vi "Generador_Entorno(SubVi).vi"(9 "Objetos":path=path "C:/Users/LuisFernando/Documents/UPIITA/8vo semestre/Instrumentacion Virtual Aplicada/Solidworks/2_Ejes_Figuras/Figuras", 10 "Mundo":path=path "C:/Users/LuisFernando/Documents/UPIITA/8vo semestre/Instrumentacion Virtual Aplicada/Solidworks/2_Ejes_Figuras/Mundo.wrl", 11 "Cluster Inicial":T1={"Opción X"=0, "Opción Y"=0, "Opción Z"=0, "Posición X"=0.0, "Velocidad X"=0.0, "Posición Y"=0.0, "Velocidad Y"=0.0, "Posición Z"=0.0, "Velocidad Z"=0.0, "Escala"=[[1.0, 1.0, 1.0], [1.0, 1.0, 1.0], [1.0, 1.0, 1.0]], "Translación"=[[1.0, 1.0, 0.0], [0.0, 0.0, 0.0], [0.0, 0.0, 0.0]], "Rotación"=[[1.0, 0.0, 0.0, 0.0], [1.0, 0.0, 0.0, 0.0], [1.0, 0.0, 0.0, 0.0]], "Operacion SX"=enum."Escala", "Eje de la Figura SX"=enum."X", "Figura Geométrica SX"=enum."Cono", "Operacion SY"=enum."Escala", "Eje de la Figura SY"=enum."Y", "Figura Geométrica SY"=enum."Cono", "Operacion SZ"=enum."Escala", "Eje de la Figura SZ"=enum."Z", "Figura Geométrica SZ"=enum."Cono"}) -> (3 "3D Picture":refnum<vi>(3d-picture))   [LabVIEW 2017]
uses:
  2_Ejes_Figuras/Control_Opciones.ctl
  2_Ejes_Figuras/Control_Operacion.ctl
  2_Ejes_Figuras/Control_Eje_Figura.ctl
  2_Ejes_Figuras/Control_Figura.ctl
  <vilib>/picture/3D Picture Control/NI_3D Picture Control.lvlib
panel:
  in  "Stop Button":bool
  out "Archivos":i32
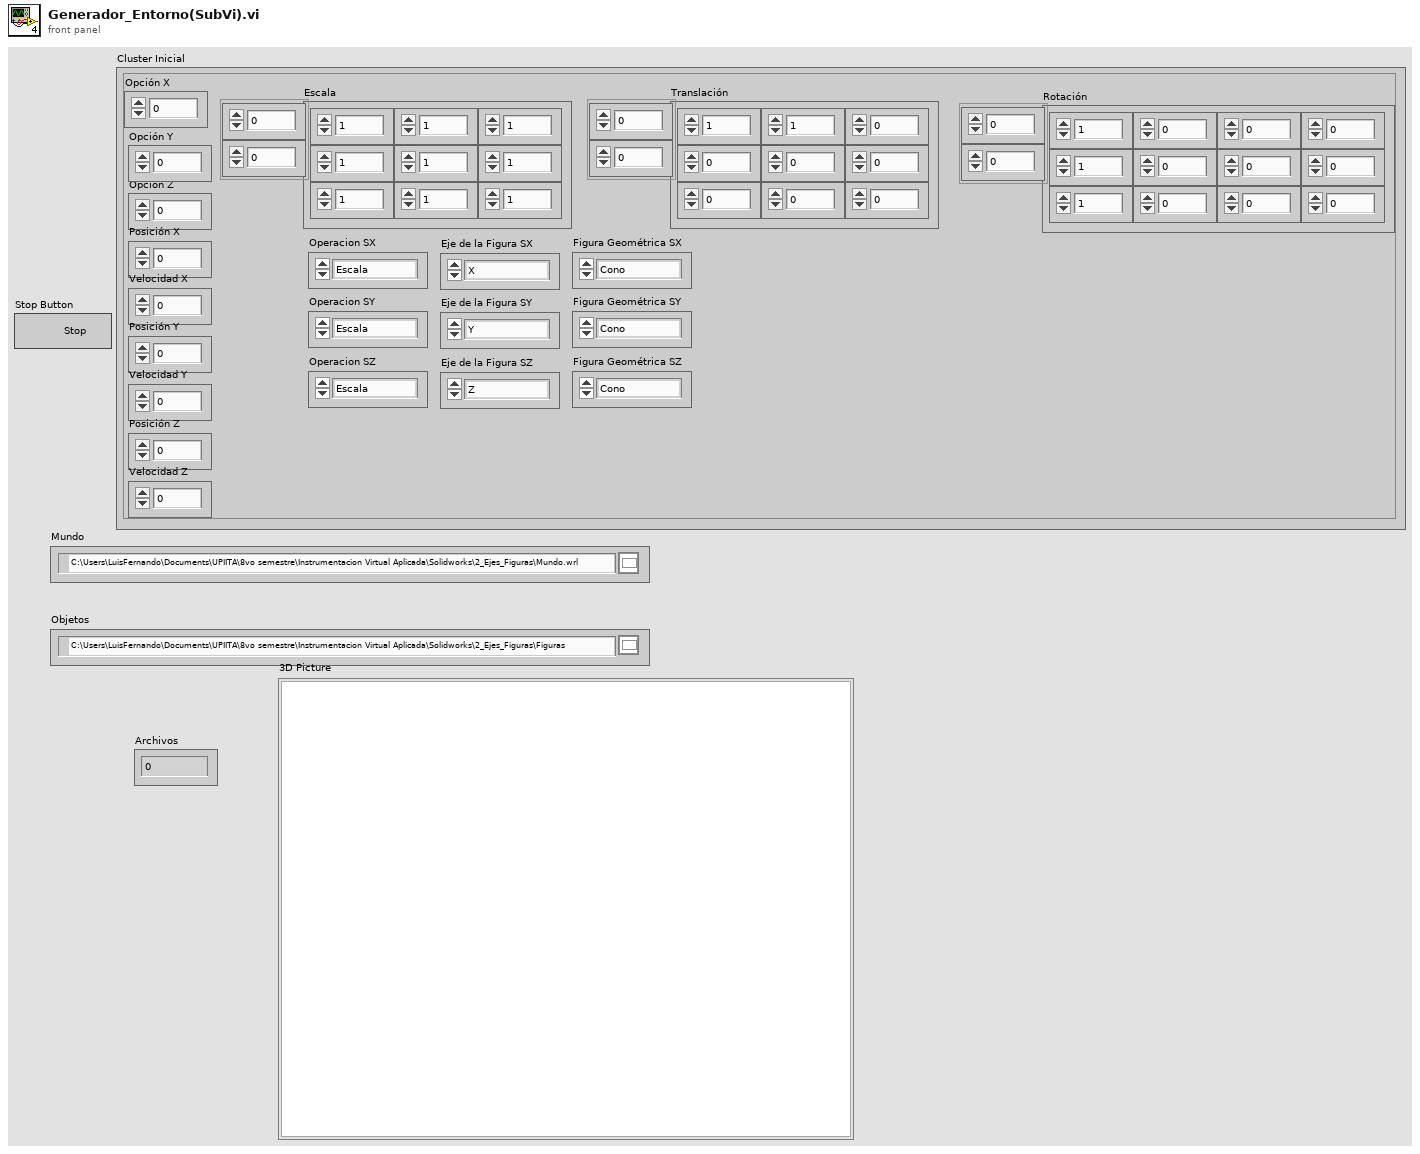
[diagram p1: front panel]
types:
  T1 = typedef "Control_Opciones.ctl" = cluster{"Opción X":i32, "Opción Y":i32, "Opción Z":i32, "Posición X":dbl, "Velocidad X":dbl, "Posición Y":dbl, "Velocidad Y":dbl, "Posición Z":dbl, "Velocidad Z":dbl, "Escala":dbl[][], "Translación":dbl[][], "Rotación":dbl[][], "Operacion SX":T2, "Eje de la Figura SX":T3, "Figura Geométrica SX":T4, "Operacion SY":T2, "Eje de la Figura SY":T3, "Figura Geométrica SY":T4, "Operacion SZ":T2, "Eje de la Figura SZ":T3, "Figura Geométrica SZ":T4}
  T2 = typedef "Control_Operacion.ctl" = enum16{"Escala", "Translación", "Rotación"}
  T3 = typedef "Control_Eje_Figura.ctl" = enum16{"X", "Y", "Z"}
  T4 = typedef "Control_Figura.ctl" = enum16{"Cono", "Esfera", "Cilindro"}
  T5 = enum16{"open", "replace", "create", "open or create", "replace or create", "replace or create with confirmation"}
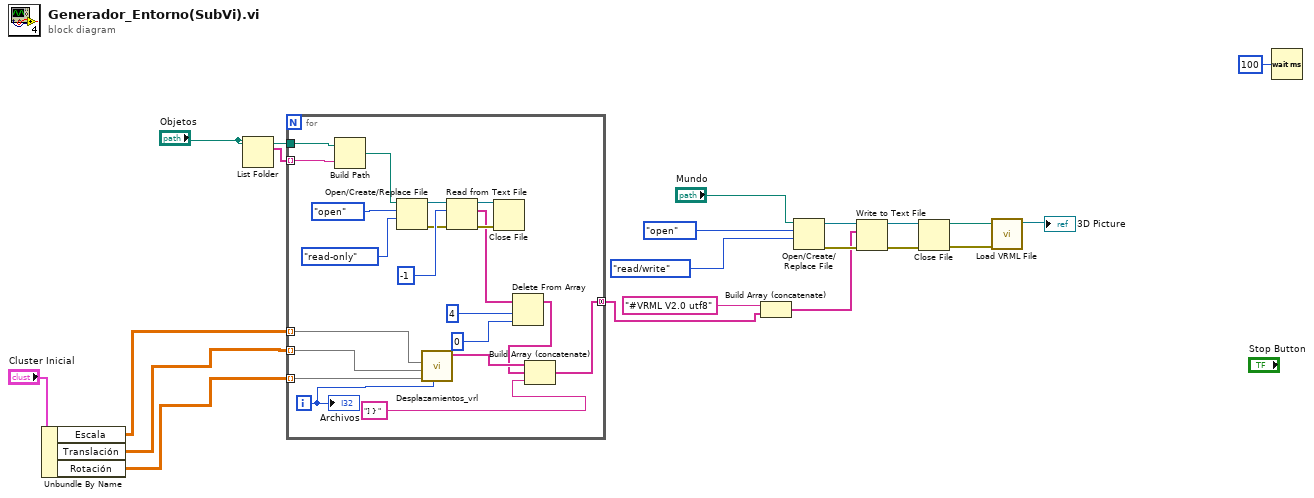
[diagram p0: block diagram]
diagram:
  n1 = Unbundle By Name("Cluster Inicial") -> ("Escala"=w3:dbl[][], "Translación"=w2:dbl[][], "Rotación"=w1:dbl[][])
  n2 = List Folder(path="Objetos") -> (filenames=w13:string[])  [unwired: 3 in, 3 out]
  n3 = for {
    tunnel: w13 -> [w41] mode=indexing
    tunnel: "Objetos" -> [w40]
    tunnel: [w24] -> w8 mode=concatenating
    tunnel: w3 -> [w28] mode=indexing
    tunnel: w2 -> [w27] mode=indexing
    tunnel: w1 -> [w26] mode=indexing
    i -> [w25]
    n4 = Build Path(base path=w40, name or relative path=w41) -> (appended path=w39:path)
    n5 = Open/Create/Replace File(file path (use dialog)=w39, operation (0:open)=T5."open", access (0:read/write)=enum16{"read/write", "read-only", "write-only"}."read-only") -> (refnum out=w36:refnum<file>, error out=w34:errorcluster)  [unwired: 3 in, 1 out]
    n6 = call "Desplazamientos_vrl.vi"("Indice"=w25, "Rotacion"=w26, "Translacion"=w27, "Escala"=w28) -> ("Salida"=w22:string[])  [unwired: 7 in]
    n7 = Read from Text File(file (use dialog)=w36, count=-1, error in=w34) -> (refnum out=w32:refnum<file>, text=w29:string[], error out=w33:errorcluster)  [unwired: 1 in, 1 out]
    n8 = Close File(refnum=w32, error in=w33) -> ()  [unwired: 2 out]
    n9 = Delete From Array(array=w29, length=4, index=0) -> (array with subset deleted=w21:string[])  [unwired: 1 out]
    n10 = Build Array (concatenate)(w22, w21, "] } ") -> (w24:string[])
    "Archivos" <- w25
  }
  n11 = Build Array (concatenate)("#VRML V2.0 utf8", w8) -> (w7:string[])
  n12 = Open/Create/Replace File(file path (use dialog)="Mundo", operation (0:open)=T5."open", access (0:read/write)=enum16{"read/write", "read-only", "write-only"}."read/write") -> (refnum out=w17:refnum<file>, error out=w16:errorcluster)  [unwired: 3 in, 1 out]
  n13 = Write to Text File(file (use dialog)=w17, text=w7, error in=w16) -> (refnum out=w14:refnum<file>, error out=w15:errorcluster)  [unwired: 1 in, 1 out]
  n14 = Close File(refnum=w14, error in=w15) -> (path=w11:path, error out=w10:errorcluster)
  n15 = call <vilib>:"Load VRML File.vi"("error in"=w10, "Path"=w11) -> ("Scene:Read Scene File"=→"3D Picture":refnum<vi>)  [unwired: 8 in, 1 out]
  n16 = Wait (ms)(milliseconds to wait=u32 100) -> ()  [unwired: 1 out]
